vi "Data to IEnum.vi"(0 "Data String In":string, 11 "error in":errorcluster) -> (4 "Data IEnum Out":refnum<k24>, 15 "error out":errorcluster)   [LabVIEW 2014, in "GEA2_Toolkit.lvlib"]
uses:
  library/GEA2_Toolkit.lvlib
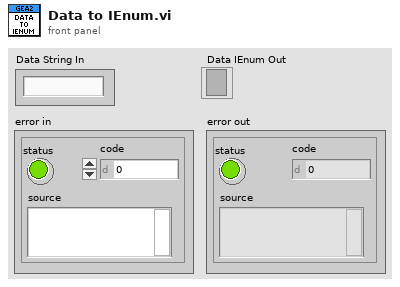
[diagram p1: front panel]
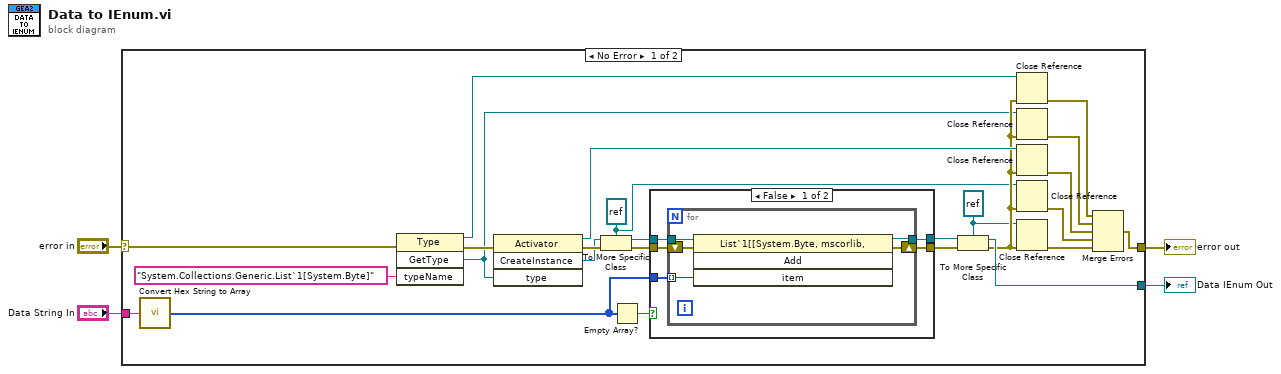
[diagram p0: block diagram]
diagram:
  n1 = case shown="No Error" "error in" {
    selector: "error in" -> [w21 w42]
    tunnel: [w20 _] -> w4
    tunnel: [w11 w42] -> w3
    tunnel: "Data String In" -> [w24 _]
    frame No Error {
      w7 = refnum<k24> refnum ("reference")
      w8 = refnum<k24> refnum ("reference")
      n2 = call "Convert Hex String to Array.vi"("Hex String In"=w24) -> ("Hex Array Out"=w18:u8[])  [unwired: 14 in]
      n3 = invoke class="Type" method="GetType"(error in=w21, "typeName"="System.Collections.Generic.List`1[System.Byte]") -> (reference out=w22:refnum<k24>, error out=w29:errorcluster, "GetType"=w10:refnum<k24>)  [unwired: 2 in, 1 out]
      n4 = invoke class="Activator" method="CreateInstance"(error in=w29, "type"=w10) -> (reference out=w23:refnum<k24>, error out=w27:errorcluster, "CreateInstance"=w9:refnum<k24>)  [unwired: 2 in, 1 out]
      n5 = To More Specific Class(target class=w8, reference=w9, error in=w27) -> (specific class reference=w26:refnum<k24>, error out=w25:errorcluster)
      n6 = Empty Array?(array=w18) -> (empty?=w17:bool)
      n7 = case shown="False" w17 {
        tunnel: w26 -> [w34 w41]
        tunnel: w25 -> [w33 w40]
        tunnel: w18 -> [w32 _]
        tunnel: [w31 w41] -> w16
        tunnel: [w30 w40] -> w19
        frame False {
          n8 = for {
            tunnel: w32 -> [w38] mode=indexing
            shift-right: [w37] -> w30
            shift-left: w33 -> [w36]
            tunnel: w34 -> [w35]
            tunnel: [w39] -> w31
            n9 = invoke class="List`1[[System.Byte, mscorlib, " method="Add"(reference=w35, error in=w36, "item"=w38) -> (reference out=w39:refnum<k24>, error out=w37:errorcluster)  [unwired: 1 in, 2 out]
          }
        }
        frame True {
        }
      }
      n10 = To More Specific Class(target class=w7, reference=w16, error in=w19) -> (specific class reference=w20:refnum<k24>, error out=w15:errorcluster)
      n11 = Close Reference(reference=w22, error in (no error)=w15) -> (error out=w6:errorcluster)
      n12 = Close Reference(reference=w10, error in (no error)=w15) -> (error out=w5:errorcluster)
      n13 = Close Reference(reference=w23, error in (no error)=w15) -> (error out=w14:errorcluster)
      n14 = Close Reference(reference=w8, error in (no error)=w15) -> (error out=w13:errorcluster)
      n15 = Close Reference(reference=w7, error in (no error)=w15) -> (error out=w12:errorcluster)
      n16 = Merge Errors(w6, w5, w14, w13, w12) -> (w11:errorcluster)
    }
    frame Error {
    }
  }
  "Data IEnum Out" <- w4
  "error out" <- w3
